vi "Anritsu VNA Set Sweep Type.vi"(6 "Channel":i8=1 min=1 step=1, 7 "Anritsu VNA":T1, 8 "error in (no error)":errorcluster, 10 "Sweep Type":T2, 11 "VISA Resource Name":refnum<visa-resource-name>) -> (0 "error out":errorcluster, 3 "dup VISA Resource Name":refnum<visa-resource-name>)   [LabVIEW 2011]
doc: "This VI for the HP8753B is used to set the meausurement format."
uses:
  TypeDefs/Anritsu VNA Sweep Type.ctl
  TypeDefs/Anritsu VNA Instrument Info.ctl
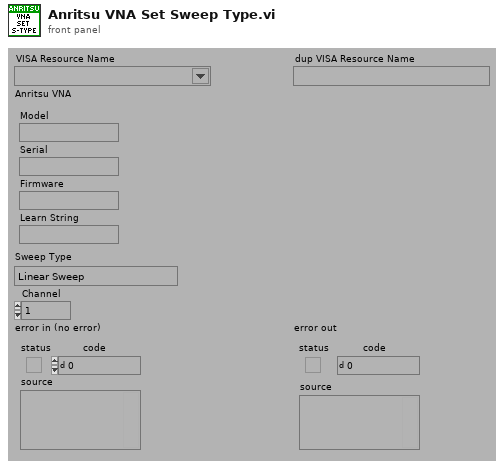
[diagram p1: front panel]
types:
  T1 = typedef "Anritsu VNA Instrument Info.ctl" = cluster{"Model":string, "Serial":string, "Firmware":string, "Learn String":string}
  T2 = typedef "Anritsu VNA Sweep Type.ctl" = enum32{"Linear Sweep", "Frequency Sweep", "Power Sweep", "CW Time Sweep", "Discrete Fill", "Time Domain", "Logarithmic Sweep", "Segmented Sweep (Frequency)", "Segmented Sweep (Index)", "MFGC"}
  T3 = typedef "Anritsu VNA Model.ctl" = enum16{"Not Supported", "37XXXX", "MS20XXX", "MS462XX", "MS464XX"}
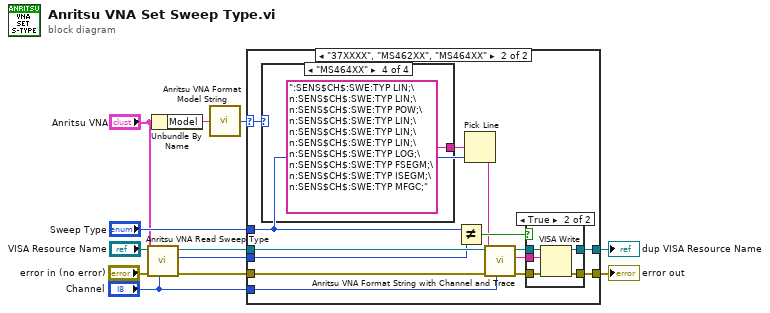
[diagram p0: block diagram]
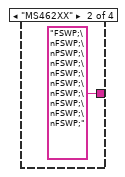
[diagram p4: hidden frame]
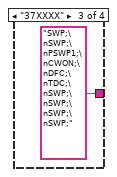
[diagram p5: hidden frame]
diagram:
  n1 = call "Anritsu VNA Read Sweep Type.vi"("Channel"="Channel", "Anritsu VNA"="Anritsu VNA", "error in (no error)"="error in (no error)", "VISA Resource Name"="VISA Resource Name") -> ("error out"=w8:errorcluster, "Sweep Type"=w5:T2, "dup VISA Resource Name"=w7:refnum<visa-resource-name>)  [unwired: 5 out]
  n2 = Unbundle By Name("Anritsu VNA") -> ("Model"=w3:string)
  n3 = call "Anritsu VNA Format Model String.vi"("Model"=w3) -> ("Model"=w2:T3)
  n4 = case shown="\"37XXXX\", \"MS462XX\", \"MS464XX\"" w2 {
    selector: w2 -> [_ w18]
    tunnel: [w14 w26] -> w12
    tunnel: [w13 w25] -> w11
    tunnel: w8 -> [w13 w24]
    tunnel: w7 -> [w14 w23]
    tunnel: "Sweep Type" -> [_ w22]
    tunnel: w5 -> [_ w21]
    tunnel: "Channel" -> [_ w15]
    frame "Not Supported", "MS20XXX" {
      # "The MS2024A, MS2026A, MS2034A, and MS2036A\nonly have the linear sweep type."
    }
    frame "37XXXX", "MS462XX", "MS464XX" {
      n5 = case shown="\"MS464XX\"" w18 {
        tunnel: [_ "FSWP;\nFSWP;\nPSWP;\nFSWP;\nFSWP;\nFSWP;\nFSWP;\nFSWP;\nFSWP;\nFSWP;" "SWP;\nSWP;\nPSWP1;\nCWON;\nDFC;\nTDC;\nSWP;\nSWP;\nSWP;\nSWP;" ":SENS$CH$:SWE:TYP LIN;\n:SENS$CH$:SWE:TYP LIN;\n:SENS$CH$:SWE:TYP POW;\n:SENS$CH$:SWE:TYP LIN;\n:SENS$CH$:SWE:TYP LIN;\n:SENS$CH$:SWE:TYP LIN;\n:SENS$CH$:SWE:TYP LOG;\n:SENS$CH$:SWE:TYP FSEGM;\n:SENS$CH$:SWE:TYP ISEGM;\n:SENS$CH$:SWE:TYP MFGC;"] -> w19
        frame "Not Supported", "MS20XXX" {
        }
        frame "MS462XX" {
        }
        frame "37XXXX" {
        }
        frame "MS464XX" {
        }
      }
      n6 = Not Equal?(x=w22, y=w21) -> (x != y?=w20:bool)
      n7 = Pick Line(multi-line string=w19, line index=w22) -> (output string=w16:string)  [unwired: 1 out]
      n8 = call "Anritsu VNA Format String with Channel and Trace.vi"("Channel"=w15, "String"=w16) -> ("String Out"=w17:string)  [unwired: 1 in, 6 out]
      n9 = case shown="True" w20 {
        tunnel: [w31 w36] -> w26
        tunnel: [w30 w35] -> w25
        tunnel: w17 -> [_ w34]
        tunnel: w24 -> [w30 w33]
        tunnel: w23 -> [w31 w32]
        frame False {
        }
        frame True {
          n10 = VISA Write(VISA resource name=w32, write buffer=w34, error in (no error)=w33) -> (VISA resource name out=w36:refnum<visa-resource-name>, error out=w35:errorcluster)  [unwired: 1 out]
        }
      }
    }
  }
  "dup VISA Resource Name" <- w12
  "error out" <- w11
